vi "Fill Sylgard Dialog.vi"(7 "Console Log in":refnum<class "Console Log.lvclass">, 8 "error in":errorcluster, 11 "Potting Procedure in":refnum<class "Potting Procedure.lvclass">) -> (0 "error out":errorcluster, 2 "Canceled":bool, 3 "Potting Procedure out":refnum<class "Potting Procedure.lvclass">, 5 "Console Log out":refnum<class "Console Log.lvclass">)   [LabVIEW 2017]
uses:
  Shared Components/Gantry Class/Gantry Class.lvclass
  Procedure Classes/Potting Procedure/Potting Procedure.lvclass
  Shared Components/WorkTable Class/WorkTable Class.lvclass
  Shared Components/Config Manager Class/Type Definitions/Named Position.ctl
  Procedure Classes/Potting Procedure/Type Definitions/Fill Sylgard.ctl
  Application Utilities/Console Log/Console Log.lvclass
panel:
  in  "Mixing Time":timestamp
  in  "OK Button":bool
  in  "Cancel Button":bool
  # "Now Mix some sylgard dummy!\nHere are instructions!\n    Step 1: Mix Sylgard\n    Step 2: ???\n    Step 3: Profit!\n\nIf sylgard has already been mixed, enter in the approximate time when it was mixed.\nClick \"OK\" when you are finished."
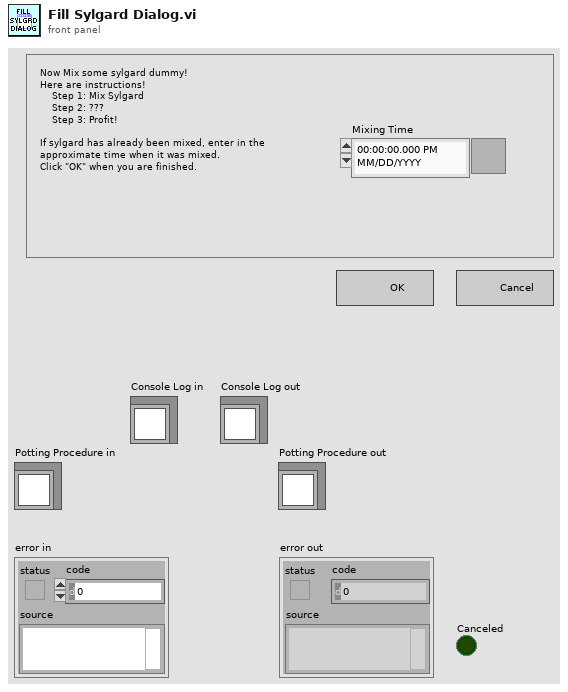
[diagram p1: front panel]
types:
  T1 = typedef "Named Position.ctl" = enum16{"home", "module_chuck_0", "module_chuck_1", "module_chuck_2", "module_chuck_3", "module_chuck_4", "glue_reservoir_chuck", "stamp_tool_chuck", "weight_tool_chuck", "needle_calibration", "tool_rack_pos_0_in", "tool_rack_pos_0_out", "tool_rack_pos_1_in", "tool_rack_pos_1_out", "tool_rack_pos_2_in", "tool_rack_pos_2_out", "front_load_position", "grabber_start_pos", "between_chuck_0_and_1", "between_chuck_2_and_3"}
  T2 = enum8{"Enabled", "Disabled", "Disabled and Grayed Out"}
  T3 = typedef "Fill Sylgard.ctl" = cluster{"Has Been Run?":bool}
  T4 = typedef "Worktable_Syringe.ctl" = cluster{"Syringe Holder":enum16{"Empty", "Populated", "Calibrated"}, "Mixing Time":timestamp, "Tip Offset":refnum<class "Vec3d Class.lvclass">}
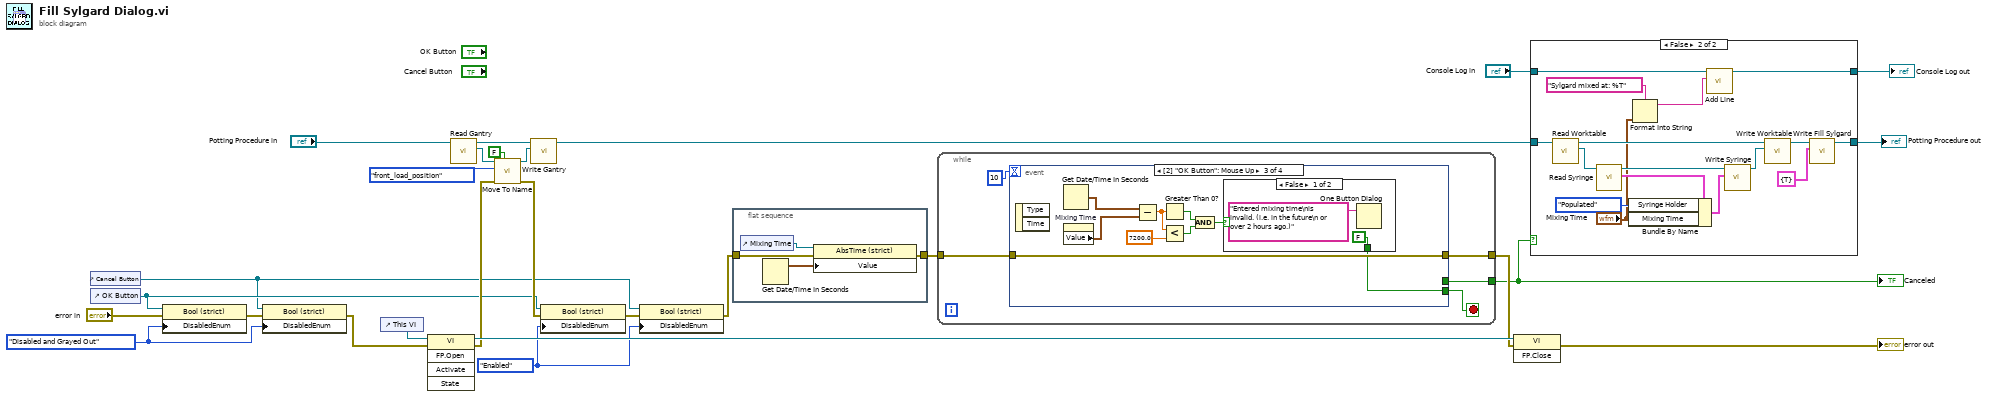
[diagram p0: block diagram]
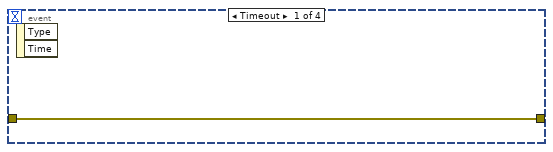
[diagram p3: hidden frame]
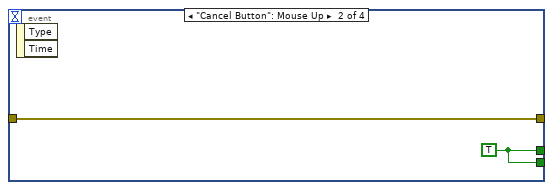
[diagram p4: hidden frame]
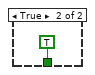
[diagram p5: hidden frame]
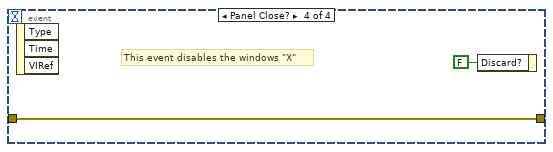
[diagram p6: hidden frame]
diagram:
  w6 = T2."Enabled" ("Disabled")
  w7 = T2."Disabled and Grayed Out" ("Disabled")
  n1 = control-ref of="Cancel Button"() -> (w8:refnum<vi>)
  n2 = control-ref of="OK Button"() -> (w9:refnum<vi>)
  n3 = property class="Bool (strict)"(reference=w9, error in="error in", "DisabledEnum"=w7) -> (error out=w13:errorcluster)  [unwired: 1 out]
  n4 = property class="Bool (strict)"(reference=w8, error in=w13, "DisabledEnum"=w7) -> (error out=w12:errorcluster)  [unwired: 1 out]
  n5 = control-ref of="This VI"() -> (w27:refnum<vi>)
  n6 = invoke class="VI" method="FP.Open"(reference=w27, error in=w12) -> (reference out=w26:refnum<vi>, error out=w20:errorcluster)  [unwired: 3 in, 3 out]
  n7 = call-dynamic "Read Gantry.vi"("Potting Procedure in"="Potting Procedure in") -> ("Gantry"=w22:refnum<class "Gantry Class.lvclass">, "Potting Procedure out"=w18:refnum<class "Potting Procedure.lvclass">)  [unwired: 8 in, 1 out]
  n8 = call-dynamic "Move To Name.vi"("Move if Same"=FALSE, "error in"=w20, "Destination"=Named_Position."front_load_position", "Gantry in"=w22) -> ("error out"=w10:errorcluster, "Gantry out"=w19:refnum<class "Gantry Class.lvclass">)  [unwired: 6 in]
  n9 = call-dynamic "Write Gantry.vi"("Gantry"=w19, "Potting Procedure in"=w18) -> ("Potting Procedure out"=w17:refnum<class "Potting Procedure.lvclass">)  [unwired: 8 in, 1 out]
  n10 = property class="Bool (strict)"(reference=w9, error in=w10, "DisabledEnum"=w6) -> (error out=w11:errorcluster)  [unwired: 1 out]
  n11 = property class="Bool (strict)"(reference=w8, error in=w11, "DisabledEnum"=w6) -> (error out=w4:errorcluster)  [unwired: 1 out]
  n12 = flat-sequence {
    tunnel: w4 -> [w29]
    tunnel: [w28] -> w3
    frame #0 {
      n13 = control-ref of="Mixing Time"() -> (w31:refnum<vi>)
      n14 = Get Date/Time In Seconds() -> (seconds since 1Jan1904=w30:timestamp)
      n15 = property class="AbsTime (strict)"(reference=w31, error in=w29, "Value"=w30) -> (error out=w28:errorcluster)  [unwired: 1 out]
    }
  }
  n16 = while {
    tunnel: [w32] -> w16
    tunnel: w3 -> [w33]
    tunnel: [w34] -> w24
    stop <- w35 stop-if-true
    n17 = event shown="[2] \"OK Button\": Mouse Up" {
      selector: _ -> [_ _ _ _]
      dyn-events: _ -> [_ _ _ _]
      timeout: 10 -> [_ _ _ _]
      tunnel: [_ w38 w40 _] -> w35
      tunnel: [w37 w39 w48 w52] -> w34
      tunnel: w33 -> [w37 w39 w48 w52]
      tunnel: [_ w38 _ _] -> w32
      event Timeout {
        n18 = event-data() -> ()  [unwired: 1 in, 2 out]
      }
      event "Cancel Button": Mouse Up {
        w38 = TRUE
        n19 = event-data() -> ()  [unwired: 1 in, 2 out]
      }
      event "OK Button": Mouse Up {
        n20 = event-data() -> ()  [unwired: 1 in, 2 out]
        n21 = Get Date/Time In Seconds() -> (seconds since 1Jan1904=w47:timestamp)
        n22 = property on="Mixing Time" class="AbsTime (strict)"() -> ("Value"=w46:timestamp)  [unwired: 2 in, 2 out]
        n23 = Subtract(x=w47, y=w46) -> (x-y=w45:dbl)
        n24 = Greater Than 0?(x=w45) -> (x > 0?=w43:bool)
        n25 = Less?(x=w45, y=7200.0) -> (x < y?=w42:bool)
        n26 = And(x=w43, y=w42) -> (x .and. y?=w41:bool)
        n27 = case shown="False" w41 {
          tunnel: [FALSE TRUE] -> w40
          frame False {
            n28 = One Button Dialog(message="Entered mixing time\nis invalid. (i.e. in the future\n or over 2 hours ago.)") -> ()  [unwired: 1 in, 1 out]
          }
          frame True {
          }
        }
      }
      event Panel Close? {
        # "This event disables the windows \"X\""
        n29 = event-data() -> ()  [unwired: 1 in, 3 out]
        n30 = event-data("Discard?"=FALSE) -> ()  [unwired: 1 in, 1 out]
      }
    }
  }
  "Canceled" <- w16
  n31 = invoke class="VI" method="FP.Close"(reference=w26, error in=w24) -> (error out=→"error out":errorcluster)  [unwired: 1 in, 2 out]
  n32 = case shown="False" w16 {
    tunnel: w17 -> [w55 w71]
    tunnel: [w55 w62] -> w15
    tunnel: "Console Log in" -> [w54 w60]
    tunnel: [w54 w59] -> w1
    frame True {
    }
    frame False {
      n33 = call-dynamic "Read Worktable.vi"("Potting Procedure in"=w71) -> ("WorkTable out"=w70:refnum<class "WorkTable Class.lvclass">, "Potting Procedure out"=w64:refnum<class "Potting Procedure.lvclass">)  [unwired: 8 in, 1 out]
      n34 = call "Read Syringe.vi"("WorkTable in"=w70) -> ("Syringe"=w69:T4, "WorkTable out"=w67:refnum<class "WorkTable Class.lvclass">)  [unwired: 8 in, 1 out]
      n35 = Bundle By Name(cluster=w69, "Syringe Holder"=enum16{"Empty", "Populated", "Calibrated"}."Populated", "Mixing Time"="Mixing Time") -> (w66:T4)
      n36 = Format Into String(format string="Sylgard mixed at: %T", "Mixing Time") -> (resulting string=w56:string)  [unwired: 2 in, 1 out]
      n37 = call "Add Line.vi"("String"=w56, "Console Log in"=w60) -> ("Console Log out"=w59:refnum<class "Console Log.lvclass">)  [unwired: 8 in, 1 out]
      n38 = call-dynamic "Write Syringe.vi"("Syringe"=w66, "WorkTable Class in"=w67) -> ("WorkTable Class out"=w65:refnum<class "WorkTable Class.lvclass">)  [unwired: 8 in, 1 out]
      n39 = call-dynamic "Write Worktable.vi"("WorkTable in"=w65, "Potting Procedure in"=w64) -> ("Potting Procedure out"=w63:refnum<class "Potting Procedure.lvclass">)  [unwired: 8 in, 1 out]
      n40 = call-dynamic "Write Fill Sylgard.vi"("Fill Sylgard"=T3 {"Has Been Run?"=TRUE}, "Potting Procedure in"=w63) -> ("Potting Procedure out"=w62:refnum<class "Potting Procedure.lvclass">)  [unwired: 8 in, 1 out]
    }
  }
  "Potting Procedure out" <- w15
  "Console Log out" <- w1
